vi "GrayOut.vi"(1 "enabled?":bool) -> (0 "state":T1(ring))   [LabVIEW 2010]
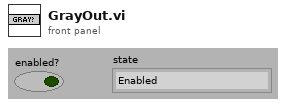
[diagram p1: front panel]
types:
  T1 = enum8{"Enabled", "Disabled", "Disabled and Grayed Out"}
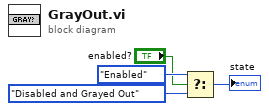
[diagram p0: block diagram]
diagram:
  n1 = Select(t=T1."Enabled" ("Disabled"), s="enabled?", f=T1."Disabled and Grayed Out" ("Disabled")) -> (s? t:f=→"state":T1)
